vi "数据写入database.vi"(9 "data输入":T1, 11 "table":string) -> (1 "error out":errorcluster)   [LabVIEW 2016, in "斯坦道CODMn.lvlib"]
uses:
  <vilib>/Utility/error.llb/DialogType.ctl
  <vilib>/addons/database/Auxilliary.llb/DB Tools Column Info.ctl
  <vilib>/addons/database/Auxilliary.llb/DB Tools DataTypes.ctl
  <vilib>/addons/database/Connection.llb/DB Tools Open Connec (String).vi
  <vilib>/addons/database/Connection.llb/Conn Execute.vi
  <vilib>/addons/database/Recordset.llb/Rec Destroy - Connection.vi
  <vilib>/addons/database/Recordset.llb/Rec Fetch Recordset Data (R).vi
  <vilib>/addons/database/NI_Database_API.lvlib
  <vilib>/Utility/VariantDataType/VariantType.lvlib
panel:
  out "data输出":T2
  out "为空？":bool
  in  "error in (no error)":errorcluster
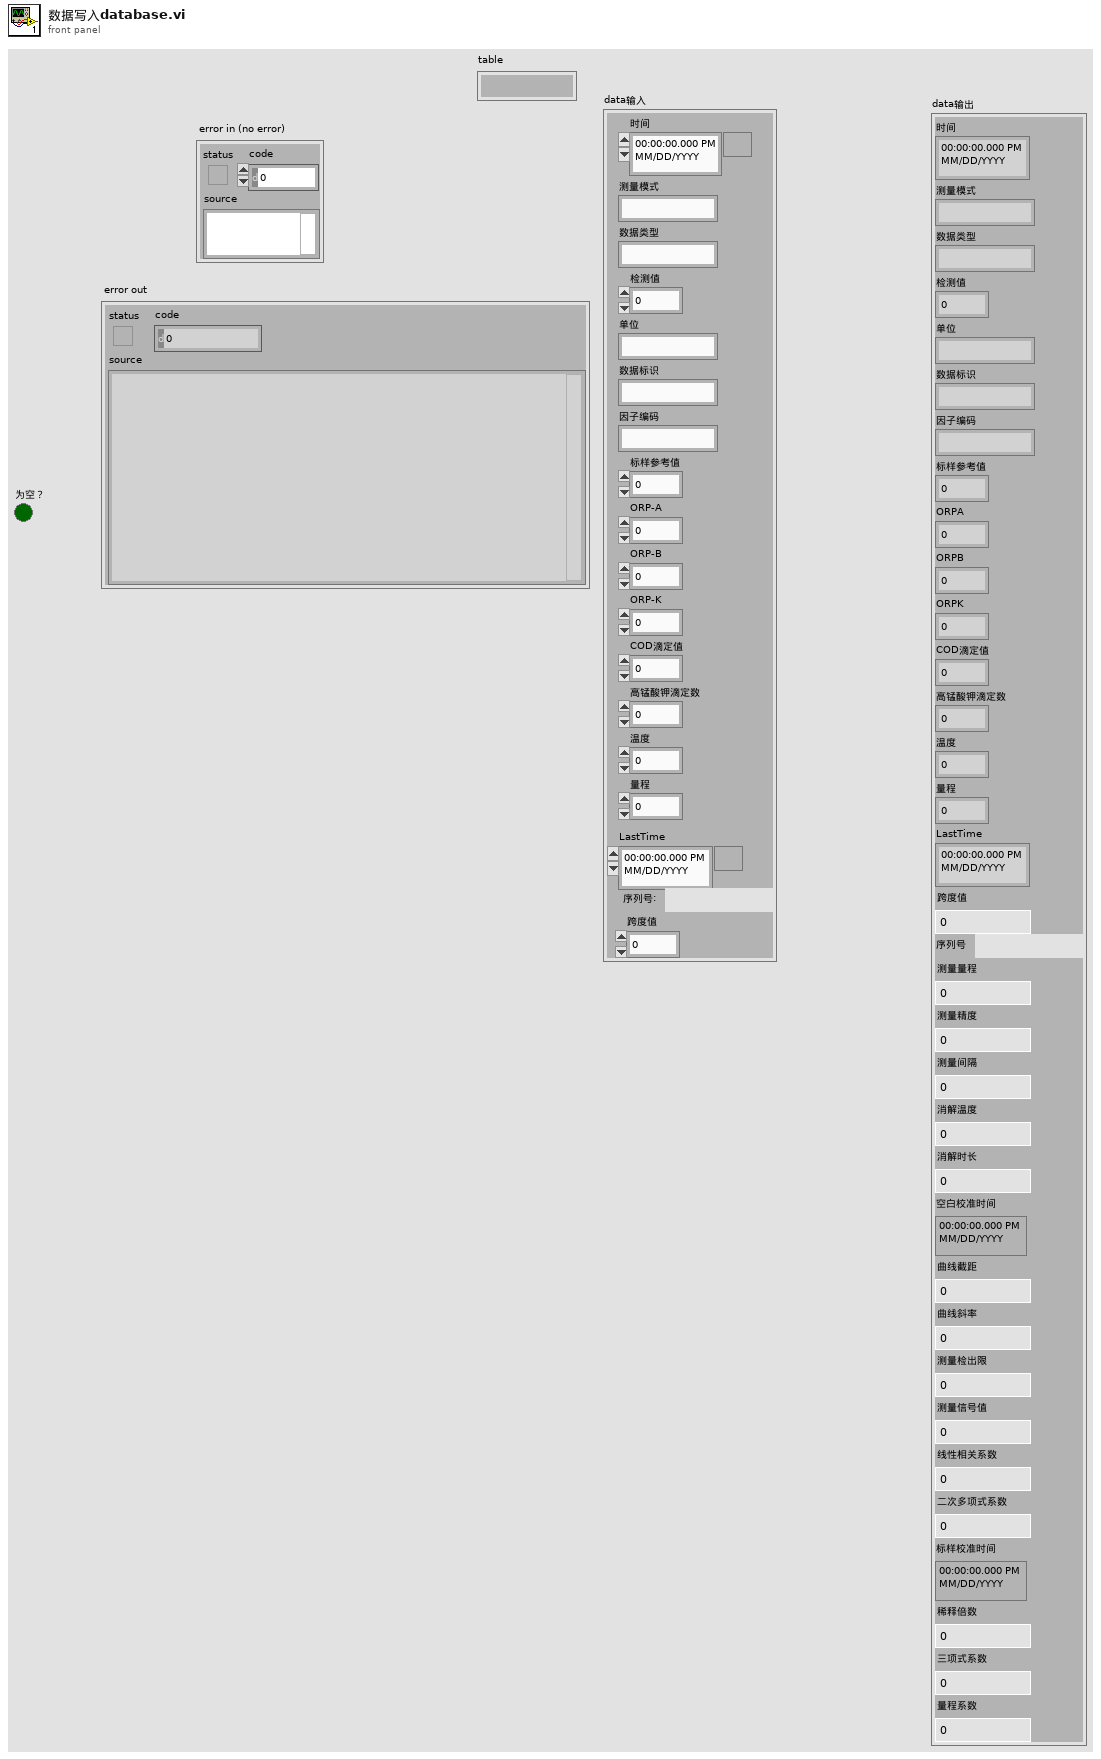
[diagram p1: front panel]
types:
  T1 = cluster{"时间":timestamp, "测量模式":string, "数据类型":string, "检测值":sgl, "单位":string, "数据标识":string, "因子编码":string, "标样参考值":sgl, "ORP-A":sgl, "ORP-B":sgl, "ORP-K":sgl, "COD滴定值":sgl, "高锰酸钾滴定数":sgl, "温度":sgl, "量程":sgl, "LastTime":timestamp, "序列号:":string, "跨度值":sgl}
  T2 = cluster{"时间":timestamp, "测量模式":string, "数据类型":string, "检测值":sgl, "单位":string, "数据标识":string, "因子编码":string, "标样参考值":sgl, "ORPA":sgl, "ORPB":sgl, "ORPK":sgl, "COD滴定值":sgl, "高锰酸钾滴定数":sgl, "温度":sgl, "量程":sgl, "LastTime":timestamp, "跨度值":sgl, "序列号":string, "测量量程":sgl, "测量精度":sgl, "测量间隔":sgl, "消解温度":sgl, "消解时长":sgl, "空白校准时间":timestamp, "曲线截距":sgl, "曲线斜率":sgl, "测量检出限":sgl, "测量信号值":sgl, "线性相关系数":sgl, "二次多项式系数":sgl, "标样校准时间":timestamp, "稀释倍数":sgl, "三项式系数":sgl, "量程系数":sgl}
  T3 = typedef "DialogType.ctl" = u16
  T4 = cluster{"测量量程":dbl, "测量精度":dbl, "测量间隔":dbl, "消解温度":dbl, "消解时长":dbl, "空白校准时间":timestamp, "曲线截距":dbl, "曲线斜率":dbl, "测量检出限":dbl, "测量信号值":dbl, "线性相关系数":dbl, "二次多项式系数":dbl, "标样校准时间":timestamp, "稀释倍数":dbl, "三项式系数":dbl, "空白标定系数":dbl, "量程系数":dbl, "F0/ORPA":dbl, "F1/ORPB":dbl, "F2/ORPK":dbl, "F3":dbl, "F4":dbl, "F5":dbl, "F6":dbl, "F7":dbl, "X0/滴定数":dbl, "量程":dbl}
  T5 = typedef "NI_Database_API.lvlib/Conn ObjectReference.ctl" = refnum<k1>
  T6 = typedef "NI_Database_API.lvlib/Rec ObjectReference.ctl" = refnum<k1>
  T7 = typedef "NI_Database_API.lvlib/DB Tools Column Info.ctl" = cluster{"column name":string, "data type":T8, "size":i32, "allow null?":bool}
  T8 = typedef "NI_Database_API.lvlib/DB Tools DataTypes.ctl" = enum16{"String", "Long (I32)", "Single (SGL)", "Double (DBL)", "Date/Time", "Binary"}
  T9 = typedef "VariantType.lvlib/Type.ctl" = enum8{"Invalid Type", "Void", "I8", "I16", "I32", "I64", "U8", "U16", "U32", "U64", "Single Float", "Double Float", "Extended Float", "Single Complex", "Double Complex", "Extended Complex", "Enum U8", "Enum U16", "Enum U32", "Enum U64", "Single Float With Unit", "Double Float With Unit", "Extended Float With Unit", "Single Complex with Unit", "Double Complex with Unit", "Extended Complex with Unit", "Boolean", "String", "Path", "Picture", "Tag", "Array", "Cluster", "Variant", "LV Variant", "Waveform", "Timestamp", "Digital Waveform", "Digital Data", "ExpressData", "Refnum", "External Data", "VI", "Poly VI", "LabVIEW Class Instance", "Fixed Point"}
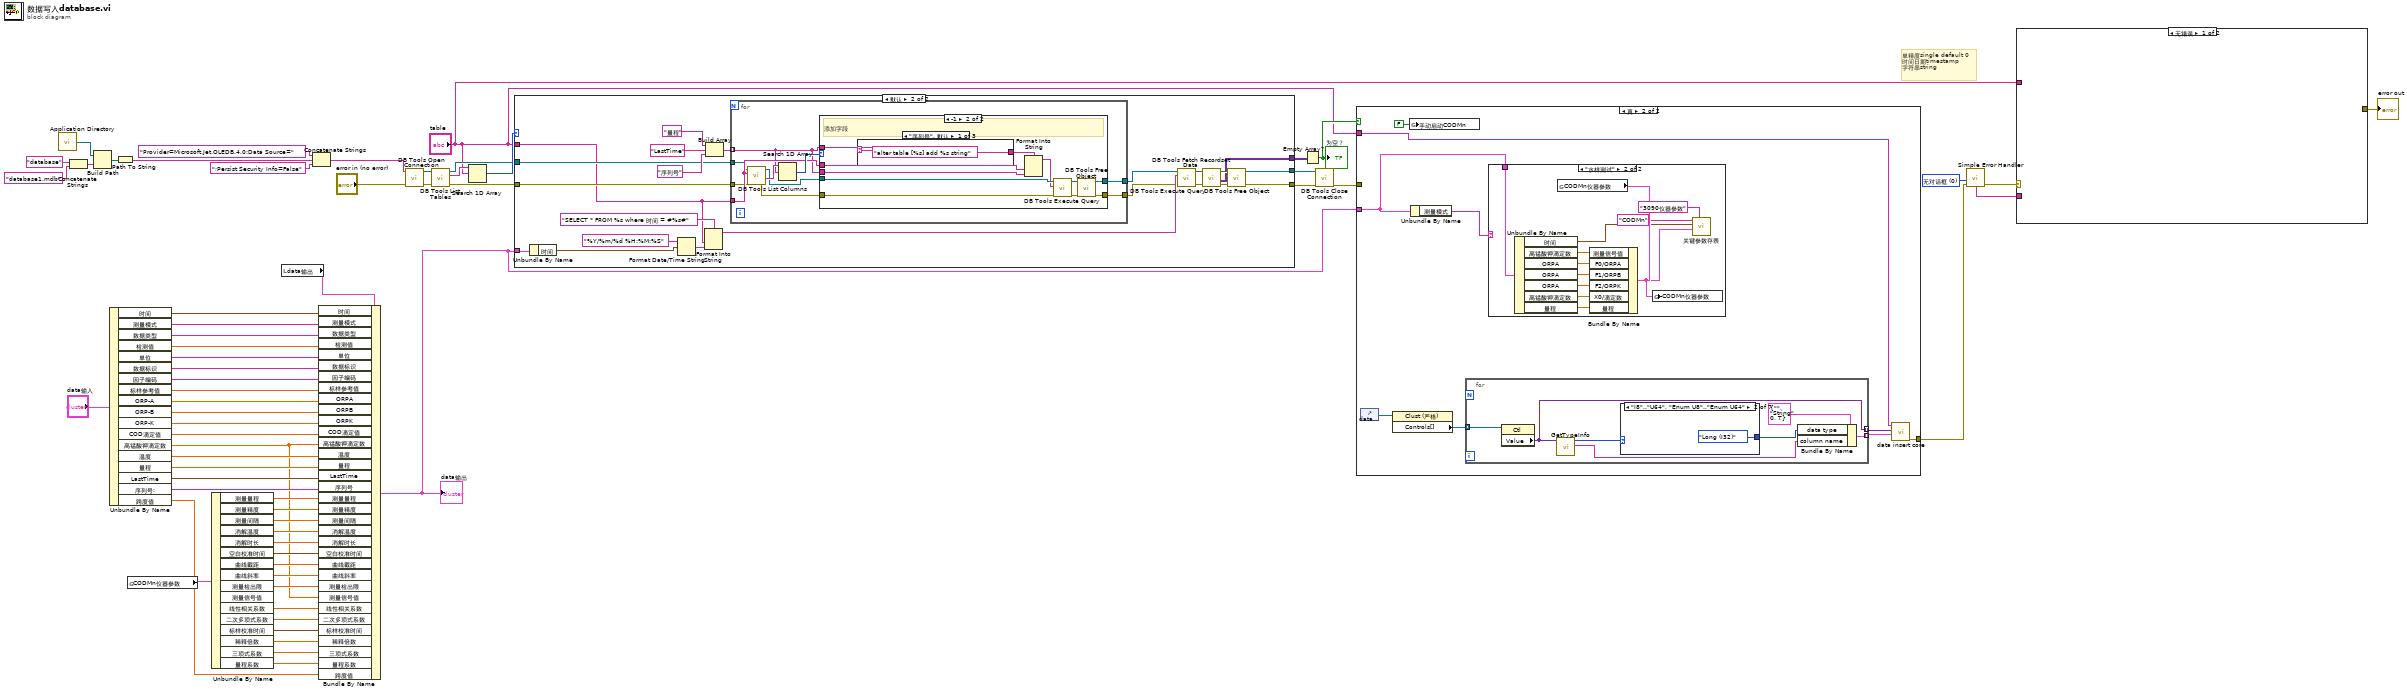
[diagram p0: block diagram]
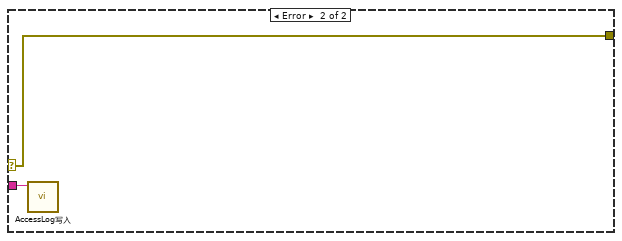
[diagram p2: hidden frame]
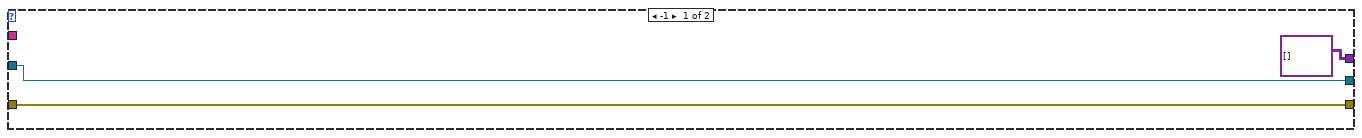
[diagram p3: hidden frame]
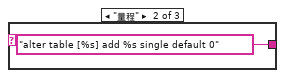
[diagram p5: hidden frame]
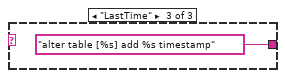
[diagram p6: hidden frame]
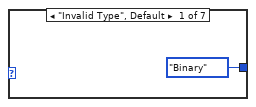
[diagram p8: hidden frame]
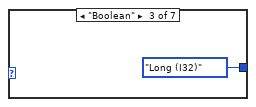
[diagram p9: hidden frame]
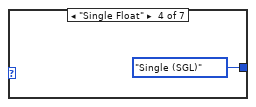
[diagram p10: hidden frame]
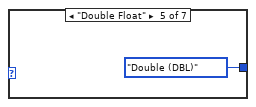
[diagram p11: hidden frame]
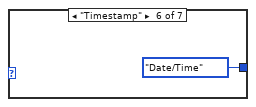
[diagram p12: hidden frame]
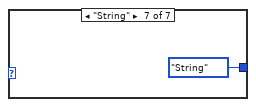
[diagram p13: hidden frame]
diagram:
  w47 = T3 0 items=["无对话框", "确定信息", "继续或停止信息", "确定信息＋警告", "继续/停止+警告"] ("type of dialog (OK msg:1)")
  # "单精度single default 0\n时间日期timestamp\n字符串string"
  n1 = call <vilib>:"Application Directory.vi"() -> ("Application Directory"=w1:path)
  n2 = Concatenate Strings("database" ("condition"), "database1.mdb" ("字符串")) -> (w58:string)
  n3 = Build Path(base path=w1, name or relative path=w58) -> (appended path=w63:path)
  n4 = Unbundle By Name("data输入") -> ("时间"=w37:timestamp, "测量模式"=w36:string, "数据类型"=w35:string, "检测值"=w34:sgl, "单位"=w33:string, "数据标识"=w32:string, "因子编码"=w31:string, "标样参考值"=w30:sgl, "ORP-A"=w29:sgl, "ORP-B"=w28:sgl, "ORP-K"=w27:sgl, "COD滴定值"=w26:sgl, "高锰酸钾滴定数"=w2:sgl, "温度"=w25:sgl, "量程"=w24:sgl, "LastTime"=w23:timestamp, "序列号:"=w22:string, "跨度值"=w5:sgl)
  n5 = Path To String(path=w63) -> (string=w62:string)
  n6 = global read "CODMn断电保存全局变量.vi" "CODMn仪器参数"() -> (w21:T4)
  n7 = Unbundle By Name(w21) -> ("测量量程"=w20:dbl, "测量精度"=w19:dbl, "测量间隔"=w18:dbl, "消解温度"=w17:dbl, "消解时长"=w16:dbl, "空白校准时间"=w15:timestamp, "曲线截距"=w14:dbl, "曲线斜率"=w13:dbl, "测量检出限"=w12:dbl, "线性相关系数"=w11:dbl, "二次多项式系数"=w10:dbl, "标样校准时间"=w9:timestamp, "稀释倍数"=w8:dbl, "三项式系数"=w7:dbl, "量程系数"=w6:dbl)  [unwired: 1 out]
  n8 = local read "data输出"() -> (w39:T2)
  n9 = Concatenate Strings("Provider=Microsoft.Jet.OLEDB.4.0;Data Source=" ("condition"), w62, ";Persist Security Info=False" ("condition")) -> (w60:string)
  n10 = Bundle By Name(cluster=w39, "时间"=w37, "测量模式"=w36, "数据类型"=w35, "检测值"=w34, "单位"=w33, "数据标识"=w32, "因子编码"=w31, "标样参考值"=w30, "ORPA"=w29, "ORPB"=w28, "ORPK"=w27, "COD滴定值"=w26, "高锰酸钾滴定数"=w2, "温度"=w25, "量程"=w24, "LastTime"=w23, "序列号"=w22, "测量量程"=w20, "测量精度"=w19, "测量间隔"=w18, "消解温度"=w17, "消解时长"=w16, "空白校准时间"=w15, "曲线截距"=w14, "曲线斜率"=w13, "测量检出限"=w12, "测量信号值"=w2, "线性相关系数"=w11, "二次多项式系数"=w10, "标样校准时间"=w9, "稀释倍数"=w8, "三项式系数"=w7, "量程系数"=w6, "跨度值"=w5) -> (w4:T2)
  "data输出" <- w4
  n11 = call-poly <vilib>:"DB Tools Open Connection.vi"("error in (no error)"="error in (no error)", "connection information"=w60) -> ("error out"=w56:errorcluster, "connection reference"=w57:T5)  [unwired: 6 in]
  n12 = call <vilib>:"DB Tools List Tables.vi"("error in (no error)"=w56, "connection reference"=w57) -> ("error out"=w52:errorcluster, "tables"=w55:string[], "connection reference out"=w53:T5)  [unwired: 3 in]
  n13 = Search 1D Array(1D array=w55, element="table") -> (index of element=w54:i32)  [unwired: 1 in]
  n14 = case shown="默认" w54 {
    tunnel: [variant[][] [] ("recordset data") w78] -> w51
    tunnel: [w67 w85] -> w42
    tunnel: [w66 w84] -> w41
    tunnel: w53 -> [w67 w72]
    tunnel: w52 -> [w66 w71]
    tunnel: "table" -> [_ w70]
    tunnel: w4 -> [_ w79]
    frame -1 {
    }
    frame Default {
      n15 = Unbundle By Name(w79) -> ("时间"=w82:timestamp)
      n16 = Format Date/Time String(time format string (%c)="%Y/%m/%d %H:%M:%S" ("时间格式字符串(%c)"), seconds (now)=w82) -> (date/time string=w80:string)  [unwired: 1 in]
      n17 = Format Into String(format string="SELECT * FROM %s where 时间 = #%s#" ("格式字符串"), w70, w80) -> (resulting string=w83:string)  [unwired: 2 in, 1 out]
      n18 = Build Array("量程" ("元素"), "LastTime" ("元素"), "序列号" ("元素")) -> (w76:string[])
      n19 = for {
        tunnel: w70 -> [w97]
        tunnel: w76 -> [w94] mode=indexing
        tunnel: [w93] -> w69
        tunnel: [w92] -> w68
        tunnel: w72 -> [w91]
        tunnel: w71 -> [w90]
        n20 = call <vilib>:"DB Tools List Columns.vi"("error in (no error)"=w90, "table"=w97, "connection reference"=w91) -> ("error out"=w95:errorcluster, "columns"=w99:string[], "connection reference out"=w96:T5)  [unwired: 1 in, 1 out]
        n21 = Search 1D Array(1D array=w99, element=w94) -> (index of element=w98:i32)  [unwired: 1 in]
        n22 = case shown="-1" w98 {
          tunnel: w96 -> [w101 w110]
          tunnel: w95 -> [w100 w109]
          tunnel: w94 -> [_ w108]
          tunnel: [w101 w106] -> w93
          tunnel: [w100 w105] -> w92
          tunnel: w97 -> [_ w104]
          tunnel: w94 -> [_ w103]
          frame 0, Default {
          }
          frame -1 {
            # "添加字段"
            n23 = case shown="\"序列号\", 默认" w103 {
              tunnel: ["alter table [%s] add %s string" "alter table [%s] add %s single default 0" "alter table [%s] add %s timestamp"] -> w102
              frame "序列号", Default {
              }
              frame "量程" {
              }
              frame "LastTime" {
              }
            }
            n24 = Format Into String(format string=w102, w104, w108) -> (resulting string=w107:string)  [unwired: 2 in, 1 out]
            n25 = call-poly <vilib>:"DB Tools Execute Query.vi"("error in (no error)"=w109, "SQL query"=w107, "connection reference"=w110) -> ("error out"=w111:errorcluster, "recordset reference"=w112:T6)  [unwired: 5 in]
            n26 = call-poly <vilib>:"DB Tools Free Object.vi"("error in (no error)"=w111, "recordset reference"=w112) -> ("error out"=w105:errorcluster, "connection reference"=w106:T5)  [unwired: 8 in]
          }
        }
      }
      n27 = call-poly <vilib>:"DB Tools Execute Query.vi"("error in (no error)"=w68, "SQL query"=w83, "connection reference"=w69) -> ("error out"=w86:errorcluster, "recordset reference"=w89:T6)  [unwired: 5 in]
      n28 = call-poly <vilib>:"DB Tools Fetch Recordset Data.vi"("error in (no error)"=w86, "recordset reference"=w89) -> ("error out"=w87:errorcluster, "recordset data"=w78:variant[][], "recordset reference out"=w88:T6)  [unwired: 3 in]
      n29 = call-poly <vilib>:"DB Tools Free Object.vi"("error in (no error)"=w87, "recordset reference"=w88) -> ("error out"=w84:errorcluster, "connection reference"=w85:T5)  [unwired: 8 in]
    }
  }
  n30 = Empty Array?(array=w51) -> (empty?=w48:bool)
  "为空？" <- w48
  n31 = call <vilib>:"DB Tools Close Connection.vi"("error in (no error)"=w41, "connection reference"=w42) -> ("error out"=w40:errorcluster)  [unwired: 5 in]
  n32 = case shown="真" w48 {
    tunnel: "table" -> [_ w117]
    tunnel: w4 -> [_ w124]
    tunnel: w40 -> [w116 _]
    tunnel: [w116 w118] -> w3
    frame False {
    }
    frame True {
      n33 = control-ref of="data输出"() -> (w121:refnum<vi>)
      n34 = property class="Clust (严格)"(reference=w121) -> ("Controls[]"=w122:refnum<vi>[])  [unwired: 1 in, 2 out]
      n35 = global write "CODMN外部API.vi" "手动启动CODMn"(FALSE ("手动启动CODMn")) -> ()
      n36 = Unbundle By Name(w124) -> ("测量模式"=w123:string)
      n37 = for {
        tunnel: w122 -> [w132] mode=indexing
        tunnel: [w126] -> w119 mode=indexing
        tunnel: [w127] -> w120 mode=indexing
        n38 = property class="Ctl"(reference=w132) -> ("Value"=w126:variant)  [unwired: 1 in, 2 out]
        n39 = call <vilib>:"GetTypeInfo.vi"("Variant"=w126) -> ("Name"=w130:string, "Type Enum"=w129:T9)  [unwired: 6 in, 3 out]
        n40 = case shown="\"I8\"..\"U64\", \"Enum U8\"..\"Enum U64\"" w129 {
          tunnel: [DB_Tools_DataTypes."Binary" ("data type") DB_Tools_DataTypes."Long (I32)" ("data type") DB_Tools_DataTypes."Long (I32)" ("data type") DB_Tools_DataTypes."Single (SGL)" ("data type") DB_Tools_DataTypes."Double (DBL)" ("data type") DB_Tools_DataTypes."Date/Time" ("data type") DB_Tools_DataTypes."String" ("data type")] -> w128
          frame "Invalid Type", Default {
          }
          frame "I8".."U64", "Enum U8".."Enum U64" {
          }
          frame "Boolean" {
          }
          frame "Single Float" {
          }
          frame "Double Float" {
          }
          frame "Timestamp" {
          }
          frame "String" {
          }
        }
        n41 = Bundle By Name(cluster=T7 {"column name"="", "data type"=enum."String", "size"=0, "allow null?"=TRUE} ("column information"), "data type"=w128, "column name"=w130) -> (w127:T7)
      }
      n42 = case shown="\"水样测试\"" w123 {
        tunnel: w124 -> [_ w150]
        frame "假", Default {
        }
        frame "水样测试" {
          n43 = Unbundle By Name(w150) -> ("时间"=w148:timestamp, "高锰酸钾滴定数"=w149:sgl, "ORPA"=w145:sgl, "ORPA"=w144:sgl, "ORPA"=w143:sgl, "高锰酸钾滴定数"=w141:sgl, "量程"=w140:sgl)
          n44 = global read "CODMn断电保存全局变量.vi" "CODMn仪器参数"() -> (w151:T4)
          n45 = Bundle By Name(cluster=w151, "测量信号值"=w149, "F0/ORPA"=w145, "F1/ORPB"=w144, "F2/ORPK"=w143, "X0/滴定数"=w141, "量程"=w140) -> (w146:T4)
          n46 = global write "CODMn断电保存全局变量.vi" "CODMn仪器参数"(w146) -> ()
          n47 = call "关键参数存表.vi"("table"="3090仪器参数", "仪器参数"=w146, "datatime"=w148, "仪器名称"="CODMn") -> ()  [unwired: 7 in, 1 out]
        }
      }
      n48 = call "data insert core.vi"("column information"=w120, "data"=w119, "table"=w117) -> ("error out"=w118:errorcluster)  [unwired: 8 in]
    }
  }
  n49 = call <vilib>:"Simple Error Handler.vi"("type of dialog (OK msg:1)"=w47, "error in (no error)"=w3) -> ("error out"=w46:errorcluster, "message"=w43:string)  [unwired: 3 in, 3 out]
  n50 = case shown="无错误" w46 {
    selector: w46 -> [_ w152]
    tunnel: "table" -> [_ _]
    tunnel: [_ w152] -> w44
    tunnel: w43 -> [_ w153]
    frame No Error {
    }
    frame Error {
      n51 = call "AccessLog写入.vi"("Log"=w153) -> ()  [unwired: 11 in]
    }
  }
  "error out" <- w44
